vi "ExposeFilterBoundControlsByRef.vi"(10 "Controls to Filter":refnum<vi>[](array[refnum]), 11 "Expose Info":T1) -> (2 "Bound Control Names":string[](array[string]), 3 "Bound Controls":refnum<vi>[](array[refnum]))   [LabVIEW 2017]
uses:
  Core/ExposeInfo.ctl
  C:/Code/CMCryoSysCode/Expose/COM/CSCom/CSCom/bin/Release/CSCom.dll
  COM/CSCom/CSCom/bin/Release/CSCom.dll
  <userlib>/_OpenG.lib/array/array.llb/Conditional Auto-Indexing Tunnel (String)__ogtk.vi
  <userlib>/_OpenG.lib/array/array.llb/Conditional Auto-Indexing Tunnel (CTL-REF)__ogtk.vi
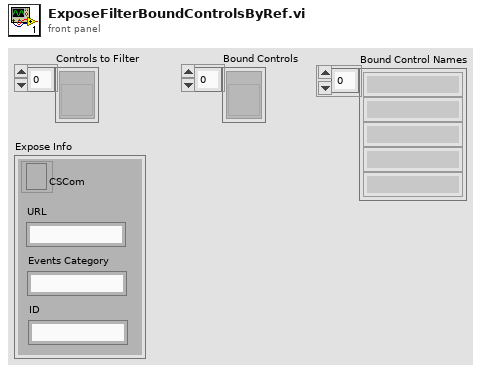
[diagram p1: front panel]
types:
  T1 = typedef "ExposeInfo.ctl" = cluster{"CSCom":refnum<k24>, "URL":string, "Events Category":string, "ID":string}
  T2 = typedef "ExposeDataType.ctl" = cluster{"Values":variant, "ParameterBindingInfo":variant}
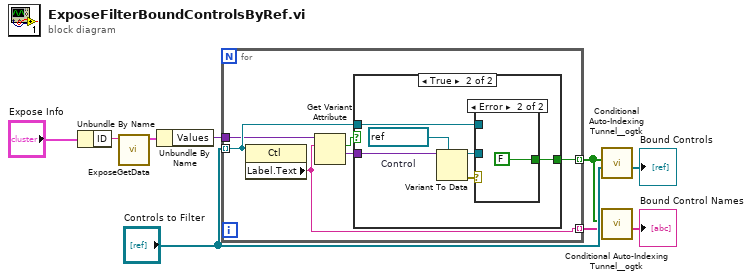
[diagram p0: block diagram]
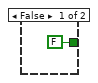
[diagram p2: hidden frame]
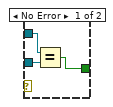
[diagram p3: hidden frame]
diagram:
  n1 = Unbundle By Name("Expose Info") -> ("ID"=w6:string)
  n2 = call "ExposeGetData.vi"("ExposeID"=w6) -> ("ExposeDataType"=w7:T2)  [unwired: 9 in, 1 out]
  n3 = Unbundle By Name(w7) -> ("Values"=w8:variant)
  n4 = for {
    tunnel: "Controls to Filter" -> [w15] mode=indexing
    tunnel: w8 -> [w14]
    tunnel: [w11] -> w2 mode=indexing
    tunnel: [w10] -> w3 mode=indexing
    n5 = property class="Ctl"(reference=w15) -> ("Label.Text"=w10:string)  [unwired: 1 in, 2 out]
    n6 = Get Variant Attribute(Variant=w14, name=w10) -> (found=w13:bool, value=w12:variant)  [unwired: 2 in, 2 out]
    n7 = case shown="True" w13 {
      tunnel: w15 -> [_ w19]
      tunnel: w12 -> [_ w21]
      tunnel: [FALSE w17] -> w11
      frame False {
      }
      frame True {
        w22 = refnum<vi> refnum  # Control
        n8 = Variant To Data(type=w22, Variant=w21) -> (data=w18:refnum<vi>, error out=w20:errorcluster)  [unwired: 1 in]
        n9 = case shown="Error" w20 {
          tunnel: w19 -> [w25 _]
          tunnel: w18 -> [w24 _]
          tunnel: [w23 FALSE] -> w17
          frame No Error {
            n10 = Equal?(x=w25, y=w24) -> (x = y?=w23:bool)
          }
          frame Error {
          }
        }
      }
    }
  }
  n11 = call-poly <userlib>:"Conditional Auto-Indexing Tunnel__ogtk.vi"("Array in"="Controls to Filter", "Elements to keep"=w2) -> ("Filtered Array out"=→"Bound Controls":refnum<vi>[])  [unwired: 5 in]
  n12 = call-poly <userlib>:"Conditional Auto-Indexing Tunnel__ogtk.vi"("Array in"=w3, "Elements to keep"=w2) -> ("Filtered Array out"=→"Bound Control Names":string[])  [unwired: 5 in]
